vi "from string.vi"(8 "error in":errorcluster, 9 "data":string, 10 "version":string, 11 "CVT configuration in":refnum<class "testmod configuration.lvclass">) -> (0 "error out":errorcluster, 3 "CVT configuration out":refnum<class "testmod configuration.lvclass">)   [LabVIEW 2013, in "testmod configuration.lvclass"]
doc: "Provides an interface for loading a module configuration from a file or other serialized data source. It is recommended that all children of this class store data in two sets--data required for its own initialization, and any data required for parent initialization--and that each implementation uses the <b>Call Parent Method</b> primitive to de-serialize parent information. As a result, it is expected that every module configuration class calls <b>component configuration.lvclass:From String.vi</b>."
uses:
  testmod configuration.lvclass
  <vilib>/NI/Tag Bus Module Framework/root configuration/TBM configuration.lvclass
  <vilib>/NI/Tag Bus Module Framework/module configuration/TBM module configuration.lvclass
  <vilib>/NI/Tag Bus Module Framework/channel/TBM channel.lvclass
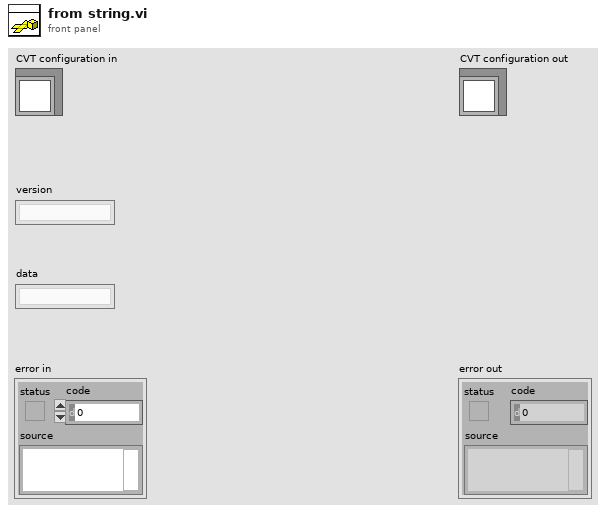
[diagram p1: front panel]
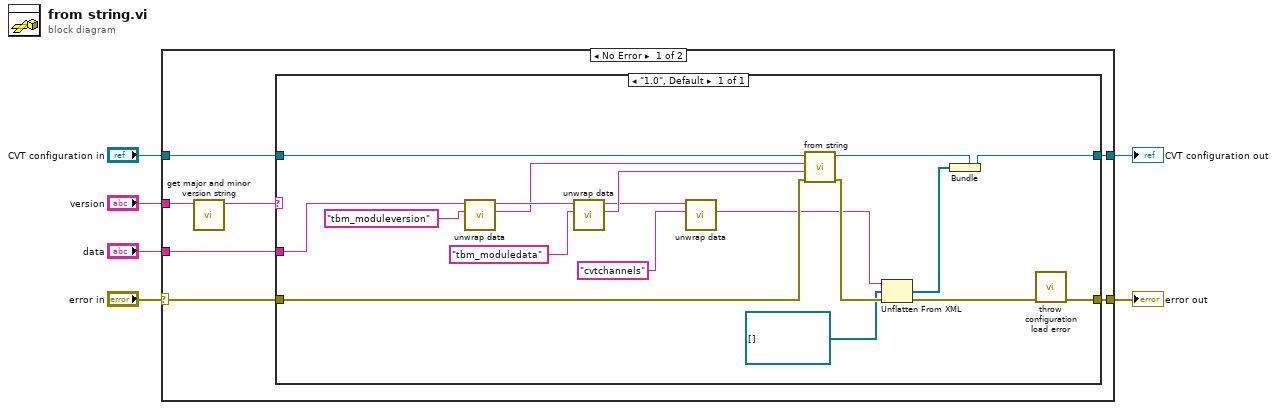
[diagram p0: block diagram]
diagram:
  n1 = case shown="No Error" "error in" {
    selector: "error in" -> [w7 w33]
    tunnel: "data" -> [w13 _]
    tunnel: "CVT configuration in" -> [w12 w32]
    tunnel: [w11 w32] -> w5
    tunnel: [w10 w33] -> w4
    tunnel: "version" -> [w9 _]
    frame No Error {
      n2 = call <vilib>:"get major and minor version string.vi"("full version"=w9) -> ("major.minor version"=w8:string)  [unwired: 10 in]
      n3 = case shown="\"1.0\", Default" w8 {
        tunnel: w13 -> [w26]
        tunnel: w7 -> [w25]
        tunnel: w12 -> [w31]
        tunnel: [w20] -> w11
        tunnel: [w28] -> w10
        frame "1.0", Default {
          n4 = call <vilib>:"unwrap data.vi"("identifier"="tbm_moduleversion" ("additional identifier"), "data to unwrap"=w26) -> ("unwrapped data"=w21:string, "remaining string"=w27:string)  [unwired: 8 in]
          n5 = call <vilib>:"unwrap data.vi"("identifier"="tbm_moduledata" ("additional identifier"), "data to unwrap"=w27) -> ("unwrapped data"=w23:string, "remaining string"=w16:string)  [unwired: 8 in]
          n6 = call <vilib>:"unwrap data.vi"("identifier"="cvtchannels" ("additional identifier"), "data to unwrap"=w16) -> ("unwrapped data"=w14:string)  [unwired: 8 in, 1 out]
          n7 = call-parent "from string.vi"("error in"=w25, "data"=w23, "version"=w21, "module configuration in"=w31) -> ("error out"=w29:errorcluster, "module configuration out"=w30:refnum<class "testmod configuration.lvclass">)  [unwired: 6 in]
          n8 = Unflatten From XML(xml string=w14, type=refnum<class "TBM channel.lvclass">[] [] ("channels"), error in (no error)=w29) -> (value=w17:refnum<class "TBM channel.lvclass">[], error out=w19:errorcluster)
          n9 = Bundle(cluster=w30, w17) -> (w20:refnum<class "testmod configuration.lvclass">)
          n10 = call <vilib>:"throw configuration load error.vi"("error in"=w19) -> ("error out"=w28:errorcluster)  [unwired: 10 in]
        }
      }
    }
    frame Error {
    }
  }
  "error out" <- w4
  "CVT configuration out" <- w5
